vi "PLL -- data source -- V3.vi"(6 "set-get delay (msec)":i64, 7 "data source action":T2=enum."get", 9 "z  in (V)":cdb, 10 "Freq in (Hz)":dbl=40000.0 format="%#_13g", 11 "PLL data source":T1=enum."MFLI") -> (1 "z out (V)":cdb=0.00010527635459-2.9308681405e-05i, 2 "Freq out (Hz)":dbl=55115.2, 3 "PLL data source OUT":T1=enum."MFLI")   [LabVIEW 2018]
uses:
  PLL data source.ctl
  data source action.ctl
  publisher action.ctl
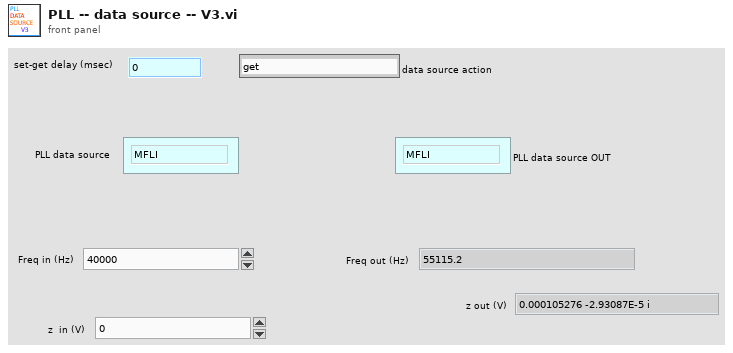
[diagram p1: front panel]
types:
  T1 = typedef "PLL data source.ctl" = enum16{"meta", "MFLI", "SRS865A"}
  T2 = typedef "data source action.ctl" = enum16{"set", "get", "init", "set-and-get", "init source"}
  T3 = typedef "publisher action.ctl" = enum16{"set", "get", "init", "check"}
  T4 = typedef "Zurich Instruments LabOne.lvlib/ziTypeHandle.ctl" = cluster{"handleValid":bool, "Conn":u64, "Path Prefix":string, "Handle":u64, "Connected":bool, "Clockbase(s)":dbl}
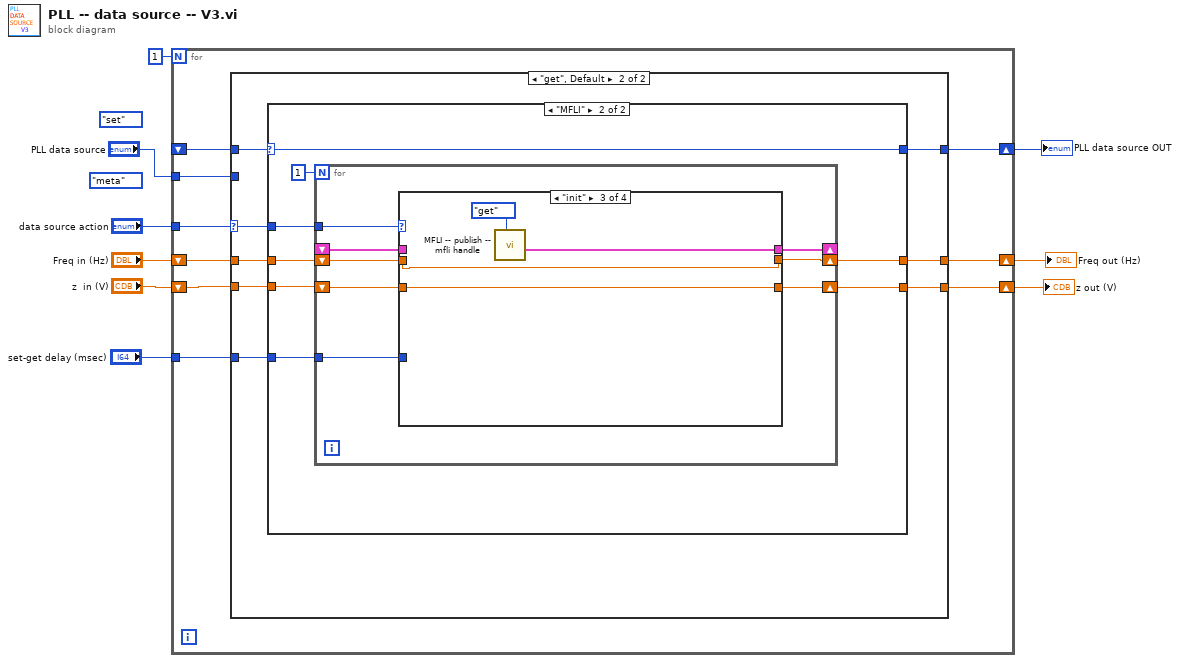
[diagram p0: block diagram]
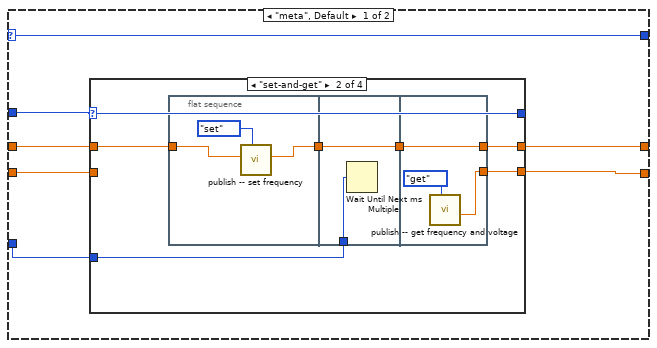
[diagram p3: hidden frame]
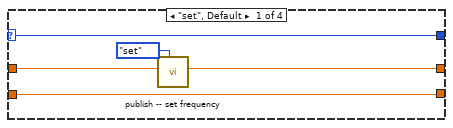
[diagram p4: hidden frame]
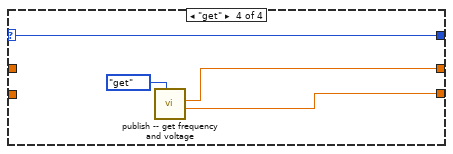
[diagram p6: hidden frame]
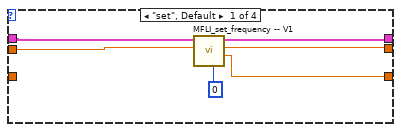
[diagram p7: hidden frame]
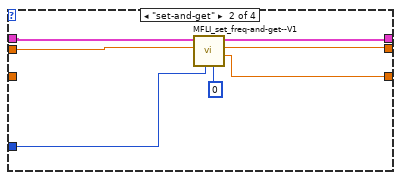
[diagram p8: hidden frame]
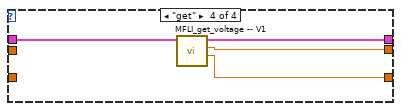
[diagram p9: hidden frame]
diagram:
  (unwired) data_source_action."set" ("data source action")
  (unwired) PLL_data_source."meta" ("PLL data source")
  n1 = for {
    N: 1 -> [_]
    tunnel: "data source action" -> [w11]
    tunnel: "set-get delay (msec)" -> [w14]
    shift-right: [w15] -> w6
    shift-left: _ -> [w18]
    shift-right: [w17] -> w8
    shift-left: "Freq in (Hz)" -> [w16]
    shift-right: [w12] -> w3
    shift-left: "z  in (V)" -> [w13]
    tunnel: "PLL data source" -> [w10]
    n2 = case shown="\"get\", Default" w11 {
      selector: w11 -> [_ w22]
      tunnel: w18 -> [_ w29]
      tunnel: [w21 w28] -> w17
      tunnel: w16 -> [w21 w27]
      tunnel: [w19 w26] -> w15
      tunnel: w14 -> [_ w25]
      tunnel: w13 -> [w20 w24]
      tunnel: [w20 w23] -> w12
      tunnel: w10 -> [w19 _]
      frame "init source" {
      }
      frame "get", Default {
        n3 = case shown="\"MFLI\"" w29 {
          selector: w29 -> [w33 w68]
          tunnel: w22 -> [w34 w67]
          tunnel: [w35 w71] -> w28
          tunnel: w27 -> [w36 w70]
          tunnel: [w33 w68] -> w26
          tunnel: w25 -> [w32 w66]
          tunnel: w24 -> [w30 w65]
          tunnel: [w31 w64] -> w23
          frame "meta", Default {
            n4 = case shown="\"set-and-get\"" w34 {
              selector: w34 -> [w38 w46 w58 w61]
              tunnel: [w39 w47 w59 w62] -> w35
              tunnel: w36 -> [w40 w48 w59 _]
              tunnel: [w38 w46 w58 w61] -> _
              tunnel: w32 -> [_ w43 _ _]
              tunnel: [w37 w42 w57 w60] -> w31
              tunnel: w30 -> [w37 _ w57 _]
              frame "set", Default {
                n5 = call "publish -- set frequency.vi"("publisher action"=publisher_action."set", "freq IN (Hz)"=w40) -> ("freq out (Hz)"=w39:dbl)  [unwired: 9 in]
              }
              frame "set-and-get" {
                n6 = flat-sequence {
                  tunnel: w48 -> [w50]
                  tunnel: [w49] -> w45
                  tunnel: w45 -> [w53]
                  tunnel: [w53] -> w44
                  tunnel: w43 -> [w52]
                  tunnel: [w56] -> w47
                  tunnel: w44 -> [w56]
                  tunnel: [w54] -> w42
                  frame #0 {
                    n7 = call "publish -- set frequency.vi"("publisher action"=publisher_action."set", "freq IN (Hz)"=w50) -> ("freq out (Hz)"=w49:dbl)  [unwired: 9 in]
                  }
                  frame #1 {
                    n8 = Wait Until Next ms Multiple(millisecond multiple=w52) -> ()  [unwired: 1 out]
                  }
                  frame #2 {
                    n9 = call "publish -- get frequency and voltage.vi"("publisher action"=publisher_action."get") -> ("Voltage out (V)"=w54:cdb)  [unwired: 8 in, 2 out]
                  }
                }
              }
              frame "init" {
              }
              frame "get" {
                n10 = call "publish -- get frequency and voltage.vi"("publisher action"=publisher_action."get") -> ("Voltage out (V)"=w60:cdb, "freq out (Hz)"=w62:dbl)  [unwired: 8 in, 1 out]
              }
            }
          }
          frame "MFLI" {
            n11 = for {
              N: 1 -> [_]
              shift-right: [w79] -> _
              shift-left: _ -> [w78]
              shift-right: [w77] -> w71
              shift-left: w70 -> [w75]
              shift-right: [w76] -> w64
              shift-left: w65 -> [w74]
              tunnel: w67 -> [w73]
              tunnel: w66 -> [w72]
              n12 = case shown="\"init\"" w73 {
                tunnel: [w85 w92 w95 w100] -> w79
                tunnel: w78 -> [w84 w91 _ w99]
                tunnel: [w81 w88 w93 w98] -> w77
                tunnel: [w80 w87 w94 w97] -> w76
                tunnel: w75 -> [w82 w89 w93 _]
                tunnel: w74 -> [_ _ w94 _]
                tunnel: w72 -> [_ w86 _ _]
                frame "set", Default {
                  n13 = call "MFLI_set_frequency -- V1.vi"("Oscillator (0)"=u16 0, "Freq in (Hz)"=w82, "Handle In"=w84) -> ("z out (V)"=w80:cdb, "Freq out (Hz)"=w81:dbl, "Handle Out"=w85:T4)  [unwired: 5 in, 1 out]
                }
                frame "set-and-get" {
                  n14 = call "MFLI_set_freq-and-get--V1.vi"("Oscillator (0)"=u16 0, "delay-circle(msec)"=w86, "Freq in (Hz)"=w89, "Handle In"=w91) -> ("z out (V)"=w87:cdb, "Freq out (Hz)"=w88:dbl, "Handle Out"=w92:T4)  [unwired: 4 in, 1 out]
                }
                frame "init" {
                  n15 = call "MFLI -- publish -- mfli handle.vi"("publisher action"=publisher_action."get") -> ("Handle Out"=w95:T4)  [unwired: 10 in]
                }
                frame "get" {
                  n16 = call "MFLI_get_voltage -- V1.vi"("Handle In"=w99) -> ("z out (V)"=w97:cdb, "Freq out (Hz)"=w98:dbl, "Handle Out"=w100:T4)  [unwired: 7 in, 1 out]
                }
              }
            }
          }
        }
      }
    }
  }
  "Freq out (Hz)" <- w8
  "z out (V)" <- w3
  "PLL data source OUT" <- w6
